vi "Word_auto_text_language.vi"(8 "error in (no error)":errorcluster, 11 "AutoTextEntries in":refnum<k7>) -> (0 "error out":errorcluster, 2 "Item out":refnum<k7>, 3 "AutoTextEntries out":refnum<k7>)   [LabVIEW 2020, in "NI_ReportGenerationToolkit.lvlib"]
uses:
  <vilib>/addons/_office/NI_ReportGenerationToolkit.lvlib
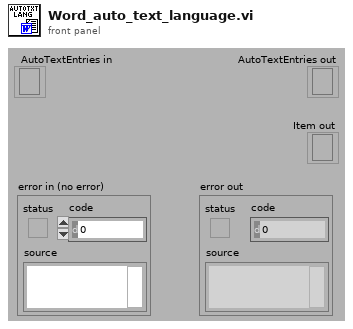
[diagram p1: front panel]
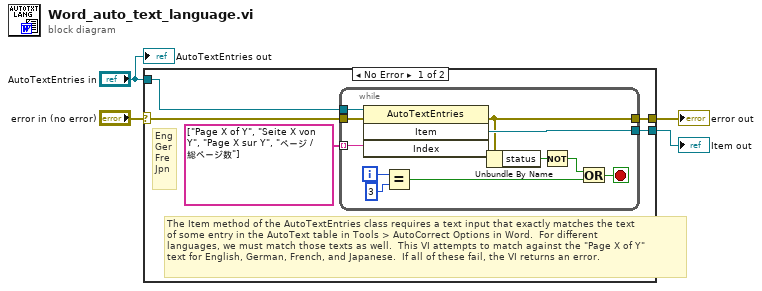
[diagram p0: block diagram]
diagram:
  n1 = case shown="No Error" "error in (no error)" {
    selector: "error in (no error)" -> [w6 w21]
    tunnel: [w9 w21] -> w4
    tunnel: "AutoTextEntries in" -> [w8 _]
    tunnel: [w7 _] -> w3
    frame No Error {
      # "The Item method of the AutoTextEntries class requires a text input that exactly matches the text\nof some entry in the AutoText table in Tools > AutoCorrect Options in Word.  For different\nlanguages, we must match those texts as well.  This VI attempts to match against the \"Page X of Y\"\ntext for English, German, French, and Japanese.  If all of these fail, the VI returns an error."
      # "Eng\nGer\nFre\nJpn"
      n2 = while {
        tunnel: [w12] -> w9
        tunnel: w8 -> [w20]
        tunnel: [w19] -> w7
        tunnel: w6 -> [w18]
        tunnel: string[] ["Page X of Y", "Seite X von Y", "Page X sur Y", "ページ / 総ページ数"] -> [w17] mode=indexing
        i -> [w15]
        stop <- w16 stop-if-true
        n3 = invoke class="AutoTextEntries" method="Item"(reference=w20, error in=w18, "Index"=w17) -> (error out=w12:errorcluster, "Item"=w19:refnum<k7>)  [unwired: 1 in, 2 out]
        n4 = Equal?(x=w15, y=3) -> (x = y?=w13:bool)
        n5 = Unbundle By Name(w12) -> ("status"=w11:bool)
        n6 = Not(x=w11) -> (.not. x?=w10:bool)
        n7 = Or(x=w10, y=w13) -> (x .or. y?=w16:bool)
      }
    }
    frame Error {
    }
  }
  "error out" <- w4
  "Item out" <- w3
  "AutoTextEntries out" <- "AutoTextEntries in"
